vi "Expand.vi"(8 "error in (no error)":errorcluster, 10 "IB_Tree.lvclass":refnum<class "IB_Tree.lvclass">, 11 "IB_TreeRootItem in":refnum<class "IB_Tree_Item_Proj_Build.lvclass">) -> (0 "error out":errorcluster, 2 "first expansion?":bool, 3 "IB_TreeRootItem out":refnum<class "IB_Tree_Item_Proj_Build.lvclass">)   [LabVIEW 2020, in "IB_Tree_Item_Proj_Build.lvclass"]
uses:
  <vilib>/AppBuilder/IB_Classes/Tree_Item_Proj_Build/IB_Tree_Item_Proj_Build.lvclass
  <vilib>/AppBuilder/IB_Classes/Tree_Item_Proj_Build/IB_Tree_Item_Proj_Build.lvclass/IB_Tree_Item_Proj_Build.ctl
  <vilib>/AppBuilder/IB_Classes/Tree_Source/IB_Tree_Source.lvclass
  <vilib>/AppBuilder/IB_Classes/Tree/IB_Tree.lvclass
  <vilib>/AppBuilder/IB_Classes/Tree_Item_Proj_Container/IB_Tree_Item_Proj_Container.lvclass
  <vilib>/AppBuilder/IB_Classes/Tree_Item_Proj_Contained_File/IB_Tree_Item_Proj_Contained_File.lvclass
  e:/builds/penguin/labview/branches/2020/dev/dist/vi.lib/AppBuilder/IB_Classes/Tree_Item_Proj_Container/IB_Tree_Item_Proj_Container.lvclass
  e:/builds/penguin/labview/branches/2020/dev/dist/vi.lib/AppBuilder/IB_Classes/Tree_Item_Proj/IB_Tree_Item_Proj.lvclass
  e:/builds/penguin/labview/branches/2020/dev/dist/vi.lib/AppBuilder/IB_Classes/Tree_Item/IB_Tree_Item.lvclass
  e:/builds/penguin/labview/branches/2020/dev/dist/vi.lib/AppBuilder/IB_Classes/Tree_Item_Proj_Build/IB_Tree_Item_Proj_Build.lvclass
  e:/builds/penguin/labview/branches/2020/dev/dist/vi.lib/AppBuilder/IB_Classes/Tree/IB_Tree.lvclass
  e:/builds/penguin/labview/branches/2020/dev/dist/vi.lib/AppBuilder/IB_Classes/Tree_Source/IB_Tree_Source.lvclass
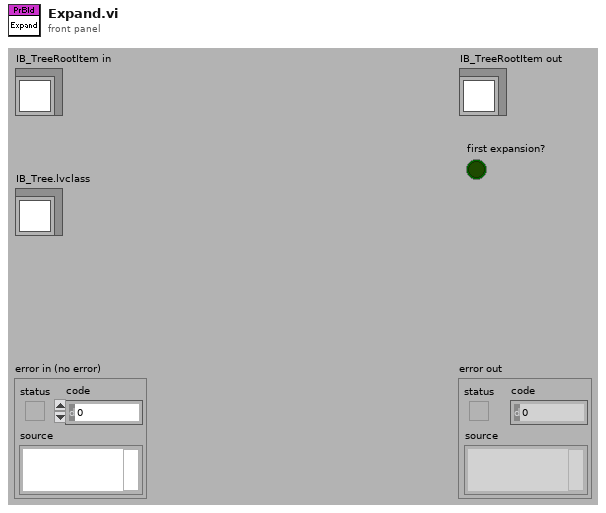
[diagram p1: front panel]
types:
  T1 = typedef "IB_Tree_Source.ctl" = cluster{"buildObject":T2}
  T2 = typedef "ItemRef.ctl" = u64
  T3 = typedef "IB_Tree_Item_Proj_Container.ctl" = cluster{"ctr files":refnum<class "IB_Tree_Item_Proj_Contained_File.lvclass">[], "previewed?":bool, "expanded?":bool, "preview error?":bool}
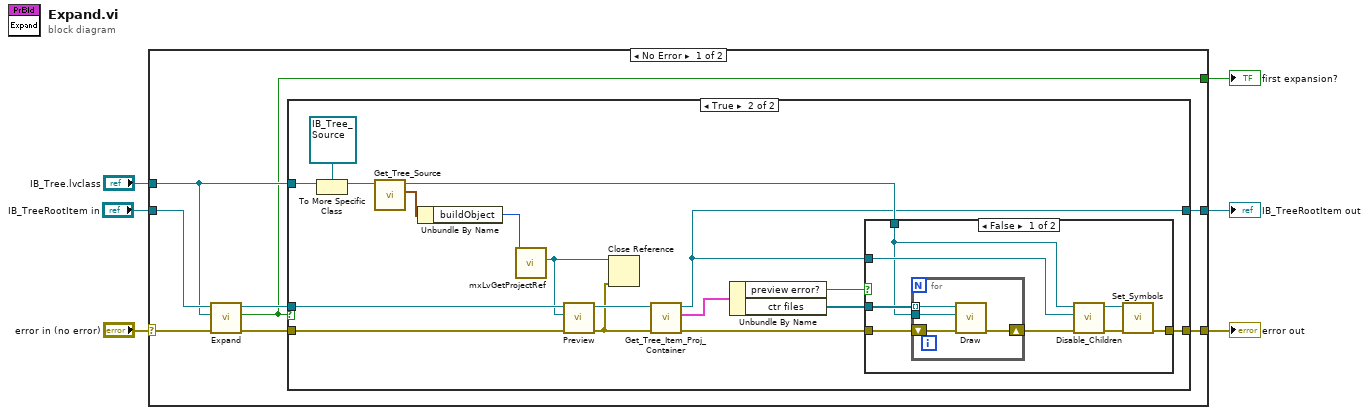
[diagram p0: block diagram]
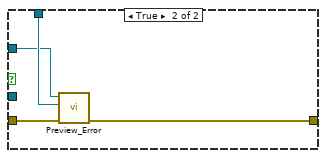
[diagram p3: hidden frame]
diagram:
  n1 = case shown="No Error" "error in (no error)" {
    selector: "error in (no error)" -> [w13 w51]
    tunnel: [w7 w51] -> w6
    tunnel: [w8 _] -> w5
    tunnel: [w10 w50] -> w4
    tunnel: "IB_Tree.lvclass" -> [w9 _]
    tunnel: "IB_TreeRootItem in" -> [w14 w50]
    frame No Error {
      n2 = call-parent "Expand.vi"("error in (no error)"=w13, "IB_Tree.lvclass"=w9, "IB_TreeRootItem in"=w14) -> ("error out"=w12:errorcluster, "first expansion?"=w8:bool, "IB_TreeRootItem out"=w11:refnum<class "IB_Tree_Item_Proj_Build.lvclass">)  [unwired: 6 out]
      n3 = case shown="True" w8 {
        tunnel: [w16 w21] -> w7
        tunnel: w12 -> [w16 w29]
        tunnel: [w15 w22] -> w10
        tunnel: w11 -> [w15 w28]
        tunnel: w9 -> [_ w33]
        frame False {
        }
        frame True {
          n4 = To More Specific Class(target class=refnum<class "IB_Tree_Source.lvclass"> refnum ("IB_SourceTree in"), reference=w33) -> (specific class reference=w32:refnum<class "IB_Tree_Source.lvclass">)  [unwired: 1 in, 1 out]
          n5 = call <vilib>:"Get_Tree_Source.vi"("IB_SourceTree in"=w32) -> ("data"=w30:T1, "IB_SourceTree out"=w27:refnum<class "IB_Tree_Source.lvclass">)  [unwired: 1 in, 8 out]
          n6 = Unbundle By Name(w30) -> ("buildObject"=w19:T2)
          n7 = call <resource>:"mxLvGetProjectRef.vi"("Item"=w19) -> ("Project Refnum"=w18:refnum<vi>)  [unwired: 8 in, 2 out]
          n8 = call-dynamic "Preview.vi"("error in (no error)"=w29, "Project"=w18, "IB_Tree_Item_Proj_Build in"=w28) -> ("error out"=w17:errorcluster, "IB_Tree_Item_Proj_Build out"=w23:refnum<class "IB_Tree_Item_Proj_Build.lvclass">)  [unwired: 7 out]
          n9 = Close Reference(reference=w18, error in (no error)=w17) -> ()  [unwired: 1 out]
          n10 = call <vilib>:"Get_Tree_Item_Proj_Container.vi"("error in (no error)"=w17, "IB_Tree_Item_Proj_Container in"=w23) -> ("error out"=w26:errorcluster, "data"=w25:T3, "IB_Tree_Item_Proj_Container out"=w22:refnum<class "IB_Tree_Item_Proj_Build.lvclass">)  [unwired: 7 out]
          n11 = Unbundle By Name(w25) -> ("preview error?"=w20:bool, "ctr files"=w24:refnum<class "IB_Tree_Item_Proj_Contained_File.lvclass">[])
          n12 = case shown="False" w20 {
            tunnel: w27 -> [w34 w49]
            tunnel: w26 -> [w38 w47]
            tunnel: w24 -> [w37 _]
            tunnel: w22 -> [w36 w48]
            tunnel: [w35 w46] -> w21
            frame False {
              n13 = for {
                tunnel: w34 -> [w45]
                shift-right: [w44] -> w39
                shift-left: w38 -> [w43]
                tunnel: w37 -> [w42] mode=indexing
                n14 = call-dynamic "Draw.vi"("error in (no error)"=w43, "IB_Tree"=w45, "IB_TreeItem in"=w42) -> ("error out"=w44:errorcluster)  [unwired: 1 in, 7 out]
              }
              n15 = call <vilib>:"Disable_Children.vi"("error in (no error)"=w39, "Tree item"=w36, "IB_Tree in"=w34) -> ("error out"=w40:errorcluster, "IB_Tree out"=w41:refnum<class "IB_Tree_Source.lvclass">)  [unwired: 7 out]
              n16 = call <vilib>:"Set_Symbols.vi"("error in (no error)"=w40, "IB_Tree in"=w41) -> ("error out"=w35:errorcluster)  [unwired: 9 out]
            }
            frame True {
              n17 = call <vilib>:"Preview_Error.vi"("error in (no error)"=w47, "IB_Tree.lvclass"=w49, "IB_Tree_Item_Proj_Container in"=w48) -> ("error out"=w46:errorcluster)  [unwired: 8 out]
            }
          }
        }
      }
    }
    frame Error {
    }
  }
  "error out" <- w6
  "IB_TreeRootItem out" <- w4
  "first expansion?" <- w5
